vi "Parse.vi"(8 "error in (no error)":errorcluster, 11 "Transform.Translate in":refnum<class "Transform.Translate.lvclass">) -> (0 "error out":errorcluster, 3 "Transform.Translate out":refnum<class "Transform.Translate.lvclass">)   [LabVIEW 2019, in "Transform.Translate.lvclass"]
uses:
  Transform.Translate.lvclass
  C:/Users/Albro/Documents/GitHub/AFM-Lithography/lvsrc/Classes/Parse/Transform/Transform.lvclass
  <vilib>/Utility/error.llb/whitespace.ctl
  Transform/Transform.lvclass/Transform.ctl
  Transform/Transform.lvclass
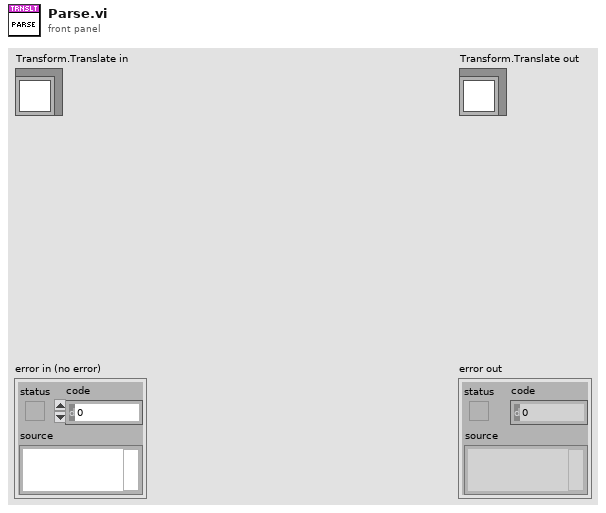
[diagram p1: front panel]
types:
  T1 = typedef "whitespace.ctl" = u16
  T2 = typedef "NI_Matrix.lvlib/RealMatrix.ctl" = dbl[][]
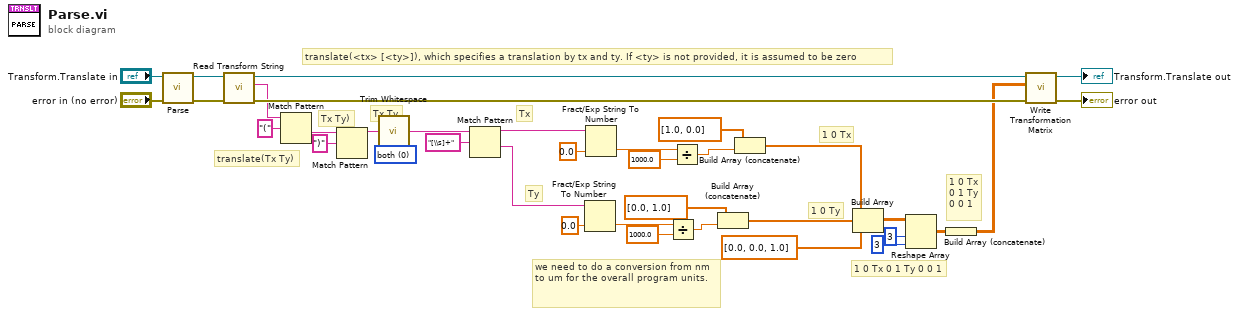
[diagram p0: block diagram]
diagram:
  w21 = T1 0 items=["both", "start of string", "end of string"] ("location (both)")
  # "we need to do a conversion from nm to um for the overall program units."
  # "translate(<tx> [<ty>]), which specifies a translation by tx and ty. If <ty> is not provided, it is assumed to be zero"
  # "1 0 Tx 0 1 Ty 0 0 1"
  # "1 0 Tx\n0 1 Ty\n0 0 1"
  # "1 0 Ty"
  # "1 0 Tx"
  # "Ty"
  # "Tx"
  # "Tx Ty"
  # "Tx Ty)"
  # "translate(Tx Ty)"
  n1 = call-parent "Parse.vi"("error in (no error)"="error in (no error)", "Transform in"="Transform.Translate in") -> ("error out"=w31:errorcluster, "Transform out"=w32:refnum<class "Transform.Translate.lvclass">)  [unwired: 8 in]
  n2 = call "Read Transform String.vi"("error in (no error)"=w31, "Transform in"=w32) -> ("error out"=w30:errorcluster, "Transform String"=w9:string, "Transform out"=w33:refnum<class "Transform.Translate.lvclass">)  [unwired: 7 in]
  n3 = Match Pattern(string=w9, regular expression="(") -> (after substring=w20:string)  [unwired: 1 in, 3 out]
  n4 = Match Pattern(string=w20, regular expression=")") -> (before substring=w26:string)  [unwired: 1 in, 3 out]
  n5 = call <vilib>:"Trim Whitespace.vi"("string"=w26, "location (both)"=w21) -> ("trimmed string"=w25:string)
  n6 = Match Pattern(string=w25, regular expression="[\\s]+") -> (before substring=w18:string, after substring=w7:string)  [unwired: 1 in, 2 out]
  n7 = Fract/Exp String To Number(string=w7, default (0 dbl)=0.0 ("default (0 DBL)")) -> (number=w3:dbl)  [unwired: 2 in, 1 out]
  n8 = Fract/Exp String To Number(string=w18, default (0 dbl)=0.0 ("default (0 DBL)")) -> (number=w5:dbl)  [unwired: 2 in, 1 out]
  n9 = Divide(x=w3, y=1000.0) -> (x/y=w2:dbl)
  n10 = Divide(x=w5, y=1000.0) -> (x/y=w4:dbl)
  n11 = Build Array (concatenate)(dbl[] [0.0, 1.0], w2) -> (w13:dbl[])
  n12 = Build Array (concatenate)(dbl[] [1.0, 0.0], w4) -> (w10:dbl[])
  n13 = Build Array(w10, w13, dbl[] [0.0, 0.0, 1.0] ("element")) -> (w12:dbl[][])
  n14 = Reshape Array(w12, 3 ("dimension size"), 3 ("dimension size")) -> (w22:dbl[][])
  n15 = Build Array (concatenate)(w22) -> (w8:T2)
  n16 = call "Write Transformation Matrix.vi"("error in (no error)"=w30, "Real Matrix"=w8, "Transform in"=w33) -> ("error out"=→"error out":errorcluster, "Transform out"=→"Transform.Translate out":refnum<class "Transform.Translate.lvclass">)  [unwired: 7 in]
